vi "Server-GUI.vi"() -> ()   [LabVIEW 2013, in "Server.lvlib" / "Server.lvclass"]
uses:
  Server.lvclass
  Supported-module-types.ctl
  Settings.ctl
panel:
  in  "Exit all clients":bool
  out "Activity log":string[](array[string])
  out "Active clients":T1(array[cluster])
  in  "Start new client":bool
  in  "Select module":T2
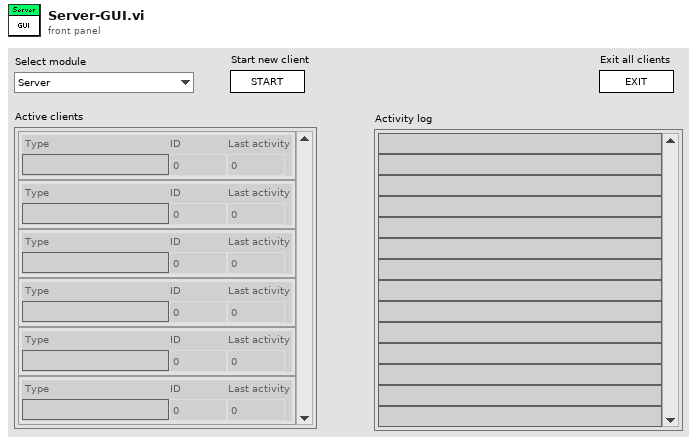
[diagram p1: front panel]
types:
  T1 = cluster{"Type":string, "ID":i32, "Last activity":i32}[]
  T2 = typedef "Server.lvlib/Server.lvclass/Supported-module-types.ctl" = enum16{"Server", "All", "BeamControl", "PowderDeposition", "StrategyParser", "CameraVision", "MaterialCharacterization", "StatusMonitor", "SLMSimulation", "LaserCharacterization"}
  T3 = typedef "Server.lvlib/Server.lvclass/Settings.ctl" = cluster{"Max clients":cluster{"Module type":T2, "MaxClients":i32, "Path":path, "Path type":bool}[], "Max backlog entries":i32, "Heartbeat timeout":dbl}
  T4 = typedef "Server.lvlib/Server.lvclass/Object-reference.ctl" = refnum<data-value>
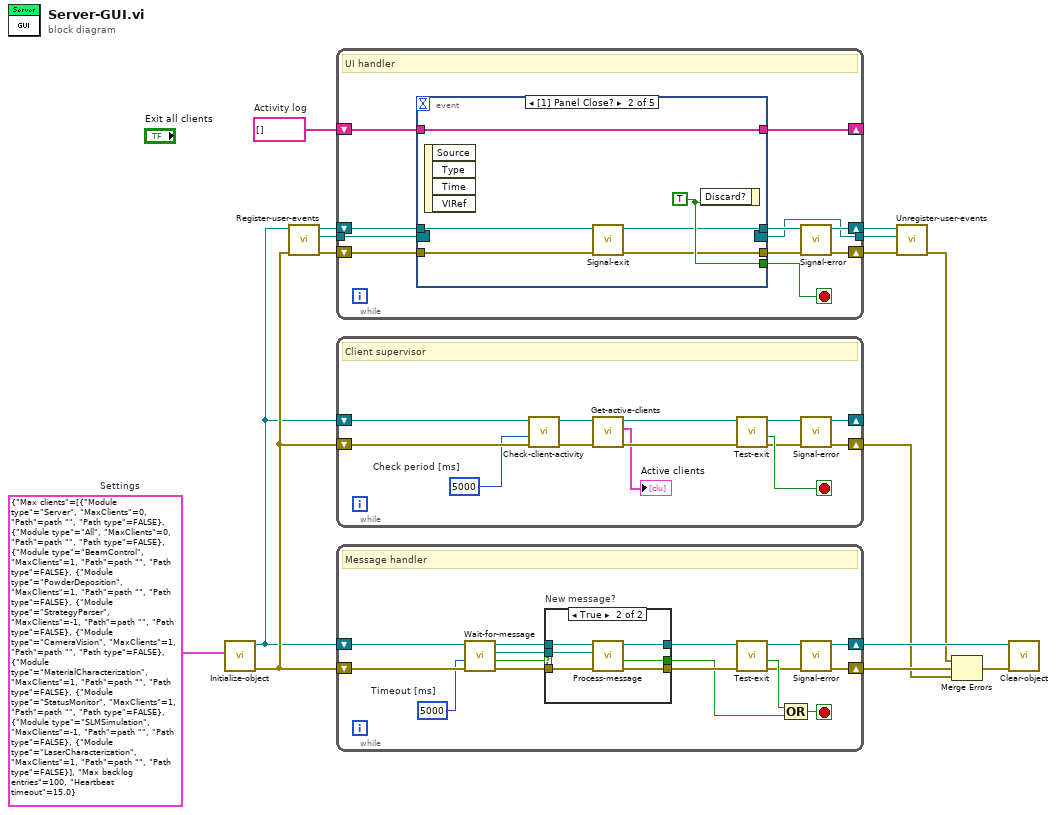
[diagram p0: block diagram]
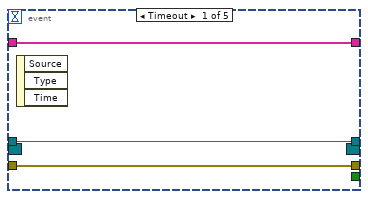
[diagram p2: hidden frame]
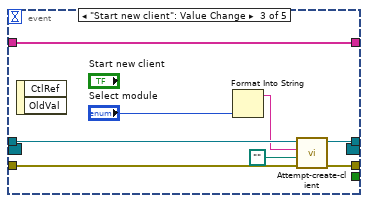
[diagram p3: hidden frame]
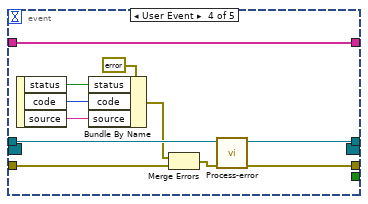
[diagram p4: hidden frame]
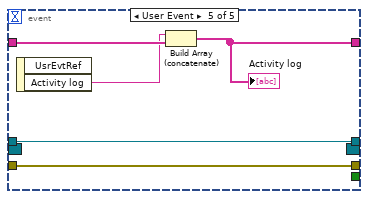
[diagram p5: hidden frame]
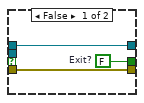
[diagram p6: hidden frame]
diagram:
  w5 = string[] []  # Activity log
  w15 = T3 {"Max clients"=[{"Module type"=enum."Server", "MaxClients"=0, "Path"=path "", "Path type"=FALSE}, {"Module type"=enum."All", "MaxClients"=0, "Path"=path "", "Path type"=FALSE}, {"Module type"=enum."BeamControl", "MaxClients"=1, "Path"=path "", "Path type"=FALSE}, {"Module type"=enum."PowderDeposition", "MaxClients"=1, "Path"=path "", "Path type"=FALSE}, {"Module type"=enum."StrategyParser", "MaxClients"=-1, "Path"=path "", "Path type"=FALSE}, {"Module type"=enum."CameraVision", "MaxClients"=1, "Path"=path "", "Path type"=FALSE}, {"Module type"=enum."MaterialCharacterization", "MaxClients"=1, "Path"=path "", "Path type"=FALSE}, {"Module type"=enum."StatusMonitor", "MaxClients"=1, "Path"=path "", "Path type"=FALSE}, {"Module type"=enum."SLMSimulation", "MaxClients"=-1, "Path"=path "", "Path type"=FALSE}, {"Module type"=enum."LaserCharacterization", "MaxClients"=1, "Path"=path "", "Path type"=FALSE}], "Max backlog entries"=100, "Heartbeat timeout"=15.0}  # Settings
  n1 = call "Initialize-object.vi"("Settings"=w15) -> ("error out"=w10:errorcluster, "Reference out"=w9:T4)  [unwired: 9 in]
  n2 = call "Register-user-events.vi"("error in (no error)"=w10, "ModComm in"=w9) -> ("error out"=w7:errorcluster, "Event Registration"=w6:refnum<event-registration>, "ModComm out"=w8:T4)  [unwired: 7 in]
  n3 = while {
    shift-right: [w19] -> w4
    shift-left: w8 -> [w25]
    shift-right: [w16] -> w3
    shift-left: w7 -> [w24]
    tunnel: w6 -> [w23]
    shift-right: [w21] -> _
    shift-left: w5 -> [w22]
    tunnel: [w18] -> w1
    stop <- w26 stop-if-true
    # "UI handler"
    n4 = event shown="[1] Panel Close?" {
      selector: w23 -> [_ _ _ _ _]
      dyn-events: [_ _ _ _ _] -> w18
      timeout: _ -> [_ _ _ _ _]
      tunnel: [_ w35 _ _ _] -> w26
      tunnel: w25 -> [w29 w34 w42 w50 w59]
      tunnel: [w29 w33 w41 w49 w59] -> w20
      tunnel: w24 -> [w28 w32 w39 w46 w58]
      tunnel: [w28 w31 w40 w45 w58] -> w17
      tunnel: w22 -> [w27 w30 w43 w44 w57]
      tunnel: [w27 w30 w43 w44 w55] -> w21
      event Timeout {
        n5 = event-data() -> ()  [unwired: 1 in, 3 out]
      }
      event Panel Close? {
        w35 = TRUE
        n6 = event-data() -> ()  [unwired: 1 in, 4 out]
        n7 = call "Signal-exit.vi"("error in (no error)"=w32, "ModComm in"=w34) -> ("error out"=w31:errorcluster, "ModComm out"=w33:T4)  [unwired: 8 in]
        n8 = event-data("Discard?"=w35) -> ()  [unwired: 1 in, 1 out]
      }
      event "Start new client": Value Change {
        n9 = event-data() -> ()  [unwired: 1 in, 2 out]
        n10 = Format Into String("Select module") -> (resulting string=w37:string)  [unwired: 3 in, 1 out]
        n11 = call "Attempt-create-client.vi"("error in (no error)"=w39, "Module path"=path "", "Module type"=w37, "ModComm in"=w42) -> ("error out"=w40:errorcluster, "ModComm out"=w41:T4)  [unwired: 6 in]
      }
      event User Event {
        n12 = event-data() -> ("status"=w53:bool, "code"=w52:i32, "source"=w51:string)  [unwired: 1 in]
        n13 = Bundle By Name(cluster=errorcluster {"status"=FALSE, "code"=0, "source"=""} ("error constant"), "status"=w53, "code"=w52, "source"=w51) -> (w47:errorcluster)
        n14 = Merge Errors(w47, w46) -> (w48:errorcluster)
        n15 = call "Process-error.vi"("error in (no error)"=w48, "ModComm in"=w50) -> ("error out"=w45:errorcluster, "ModComm out"=w49:T4)  [unwired: 8 in]
      }
      event User Event {
        n16 = event-data() -> ("Activity log"=w56:string)  [unwired: 1 in, 1 out]
        n17 = Build Array (concatenate)(w56, w57) -> (w55:string[])
        "Activity log" <- w55
      }
    }
    n18 = call "Signal-error.vi"("error in (no error)"=w17, "ModComm in"=w20) -> ("error out"=w16:errorcluster, "ModComm out"=w19:T4)  [unwired: 8 in]
  }
  n19 = while {
    shift-right: [w66] -> _
    shift-left: w9 -> [w71]
    shift-right: [w67] -> w11
    shift-left: w10 -> [w70]
    stop <- w72 stop-if-true
    w65 = u32 5000  # Check period [ms]
    # "Client supervisor"
    n20 = call "Check-client-activity.vi"("error in (no error)"=w70, "Check period"=w65, "ModComm in"=w71) -> ("error out"=w62:errorcluster, "ModComm out"=w64:T4)  [unwired: 7 in]
    n21 = call "Get-active-clients.vi"("error in (no error)"=w62, "ModComm in"=w64) -> ("error out"=w61:errorcluster, "Active clients"=→"Active clients":T1, "ModComm out"=w63:T4)  [unwired: 7 in]
    n22 = call "Test-exit.vi"("error in (no error)"=w61, "ModComm in"=w63) -> ("error out"=w68:errorcluster, "Exit?"=w72:bool, "ModComm out"=w69:T4)  [unwired: 7 in]
    n23 = call "Signal-error.vi"("error in (no error)"=w68, "ModComm in"=w69) -> ("error out"=w67:errorcluster, "ModComm out"=w66:T4)  [unwired: 8 in]
  }
  n24 = while {
    shift-right: [w74] -> w14
    shift-left: w9 -> [w88]
    shift-right: [w73] -> w13
    shift-left: w10 -> [w87]
    stop <- w79 stop-if-true
    w86 = 5000  # Timeout [ms]
    # "Message handler"
    n25 = call "Wait-for-message.vi"("error in (no error)"=w87, "Timeout"=w86, "ModComm in"=w88) -> ("error out"=w83:errorcluster, "New message?"=w85:bool, "Message"=w82:refnum<class "Message.lvclass">, "ModComm out"=w84:T4)  [unwired: 5 in]
    n26 = case "New message?" shown="True" w85 {
      tunnel: w84 -> [w91 w97]
      tunnel: w83 -> [w89 w96]
      tunnel: w82 -> [_ w95]
      tunnel: [w89 w94] -> w80
      tunnel: [w91 w93] -> w81
      tunnel: [w90 w92] -> w77
      frame False {
        w90 = FALSE  # Exit?
      }
      frame True {
        n27 = call "Process-message.vi"("error in (no error)"=w96, "Message"=w95, "ModComm in"=w97) -> ("error out"=w94:errorcluster, "Exit?"=w92:bool, "ModComm out"=w93:T4)  [unwired: 6 in]
      }
    }
    n28 = call "Test-exit.vi"("error in (no error)"=w80, "ModComm in"=w81) -> ("error out"=w76:errorcluster, "Exit?"=w78:bool, "ModComm out"=w75:T4)  [unwired: 7 in]
    n29 = Compound Arithmetic op=OR(w78, w77) -> (w79:bool)
    n30 = call "Signal-error.vi"("error in (no error)"=w76, "ModComm in"=w75) -> ("error out"=w73:errorcluster, "ModComm out"=w74:T4)  [unwired: 8 in]
  }
  n31 = call "Unregister-user-events.vi"("error in (no error)"=w3, "Event Registration"=w1, "ModComm in"=w4) -> ("error out"=w2:errorcluster)  [unwired: 7 in, 1 out]
  n32 = Merge Errors(w2, w13, w11) -> (w12:errorcluster)
  n33 = call "Clear-object.vi"("error in (no error)"=w12, "Reference in"=w14) -> ()  [unwired: 8 in, 2 out]
